vi "MEMR-Initialize Display.vi"(0 "Run":i32, 7 "State":T3, 9 "Total Nreps":i32, 11 "error in (no error)":errorcluster, 12 "Analysis":T1, 13 "controls":T2) -> (15 "error out":errorcluster)   [LabVIEW 2020]
uses:
  Typedefs/MEMR-Analysis State.ctl
  Typedefs/MEMR-Controls.ctl
  Typedefs/MEMR-Analysis.ctl
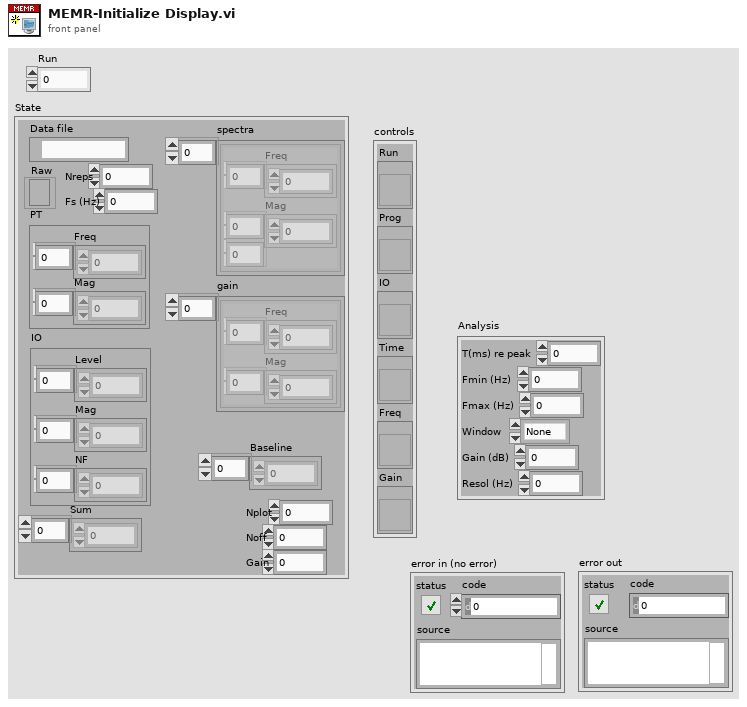
[diagram p1: front panel]
types:
  T1 = typedef "MEMR-Analysis.ctl" = cluster{"T(ms) re peak":dbl, "Fmin (Hz)":dbl, "Fmax (Hz)":dbl, "Window":enum16{"None", "Hanning", "Hamming"}, "Gain (dB)":dbl, "Resol (Hz)":dbl}
  T2 = typedef "MEMR-Controls.ctl" = cluster{"Run":refnum<vi>, "Prog":refnum<vi>, "IO":refnum<vi>, "Time":refnum<vi>, "Freq":refnum<vi>, "Gain":refnum<vi>}
  T3 = typedef "MEMR-Analysis State.ctl" = cluster{"Data file":path, "Raw":refnum<file>, "PT":cluster{"Freq":dbl[], "Mag":dbl[]}, "IO":cluster{"Level":dbl[], "Mag":dbl[], "NF":dbl[]}, "Nreps":i32, "Fs (Hz)":dbl, "Sum":dbl[], "Nplot":i32, "Noff":i32, "Gain":dbl, "spectra":cluster{"Freq":dbl[], "Mag":dbl[][]}[], "gain":cluster{"Freq":dbl[], "Mag":dbl[]}[], "Baseline":dbl[]}
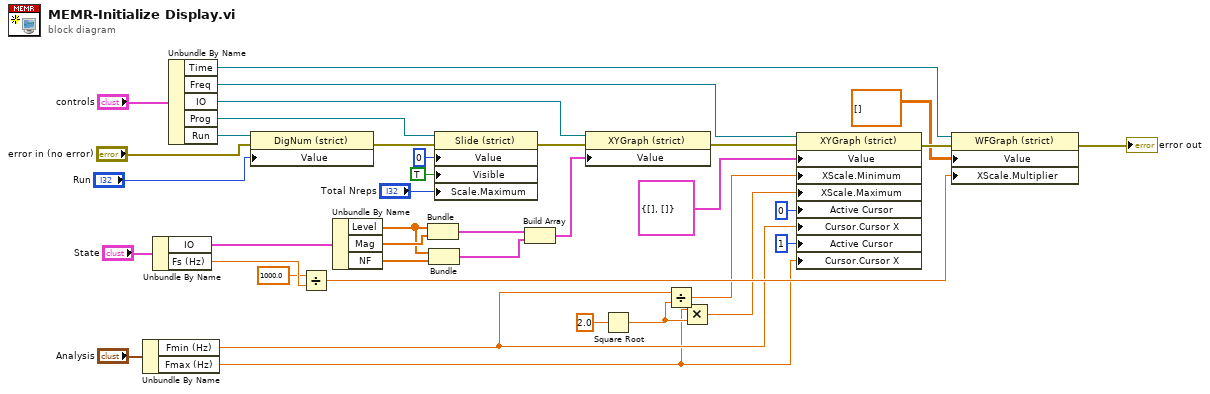
[diagram p0: block diagram]
diagram:
  n1 = Unbundle By Name("Analysis") -> ("Fmin (Hz)"=w9:dbl, "Fmax (Hz)"=w7:dbl)
  n2 = Unbundle By Name("State") -> ("IO"=w26:cluster{"Level":dbl[], "Mag":dbl[], "NF":dbl[]}, "Fs (Hz)"=w17:dbl)
  n3 = Unbundle By Name("controls") -> ("Time"=w22:refnum<vi>, "Freq"=w25:refnum<vi>, "IO"=w29:refnum<vi>, "Prog"=w35:refnum<vi>, "Run"=w37:refnum<vi>)
  n4 = property class="DigNum (strict)"(reference=w37, error in="error in (no error)", "Value"="Run") -> (error out=w34:errorcluster)  [unwired: 1 out]
  n5 = Divide(x=1000.0, y=w17) -> (x/y=w15:dbl)
  n6 = Unbundle By Name(w26) -> ("Level"=w3:dbl[], "Mag"=w4:dbl[], "NF"=w5:dbl[])
  n7 = Bundle("Level"=w3, "Mag"=w4) -> (w2:cluster{"Level":dbl[], "Mag":dbl[]})  [unwired: 1 in]
  n8 = Bundle("Level"=w3, "NF"=w5) -> (w1:cluster{"Level":dbl[], "NF":dbl[]})  [unwired: 1 in]
  n9 = property class="Slide (strict)"(reference=w35, error in=w34, "Value"=u8 0, "Visible"=TRUE, "Scale.Maximum"="Total Nreps") -> (error out=w28:errorcluster)  [unwired: 1 out]
  n10 = Build Array(w2, w1) -> (w6:cluster{"Level":dbl[], "NF":dbl[]}[])
  n11 = property class="XYGraph (strict)"(reference=w29, error in=w28, "Value"=w6) -> (error out=w24:errorcluster)  [unwired: 1 out]
  n12 = Square Root(x=2.0) -> (sqrt(x)=w11:dbl)
  n13 = Divide(x=w9, y=w11) -> (x/y=w14:dbl)
  n14 = Multiply(x=w7, y=w11) -> (x*y=w12:dbl)
  n15 = property class="XYGraph (strict)"(reference=w25, error in=w24, "Value"=cluster{dbl[], dbl[]} {[], []}, "XScale.Minimum"=w14, "XScale.Maximum"=w12, "Active Cursor"=u32 0, "Cursor.Cursor X"=w9, "Active Cursor"=u32 1, "Cursor.Cursor X"=w7) -> (error out=w21:errorcluster)  [unwired: 1 out]
  n16 = property class="WFGraph (strict)"(reference=w22, error in=w21, "Value"=dbl[][] [], "XScale.Multiplier"=w15) -> (error out=→"error out":errorcluster)  [unwired: 1 out]
